vi "DAQNavi Write (Digital Wfm 1Chan 1Samp).vi"(8 "error in (no error)":errorcluster, 9 "timeout":dbl=10.0, 10 "data":digitalwaveform(waveform)={"t0"=timestamp(0 s since 1904-01-01), "dt"=1.0, "Y"={"transitions"=[], "data"=[]}}, 11 "task in":i32) -> (0 "error out":errorcluster, 2 "number of samples written per channel":u32, 3 "task out":i32)   [LabVIEW 2020]
uses:
  <vilib>/Waveform/DWDTOps.llb/DWDT Digital to Binary U8.vi
  DAQNavi_LV.dll
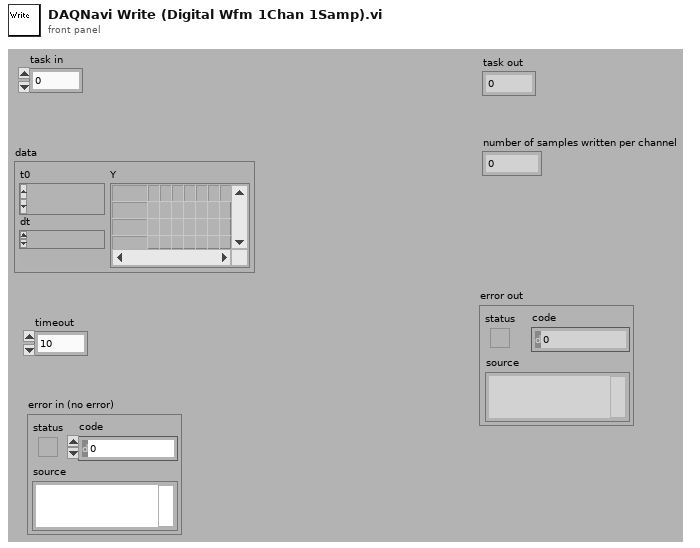
[diagram p1: front panel]
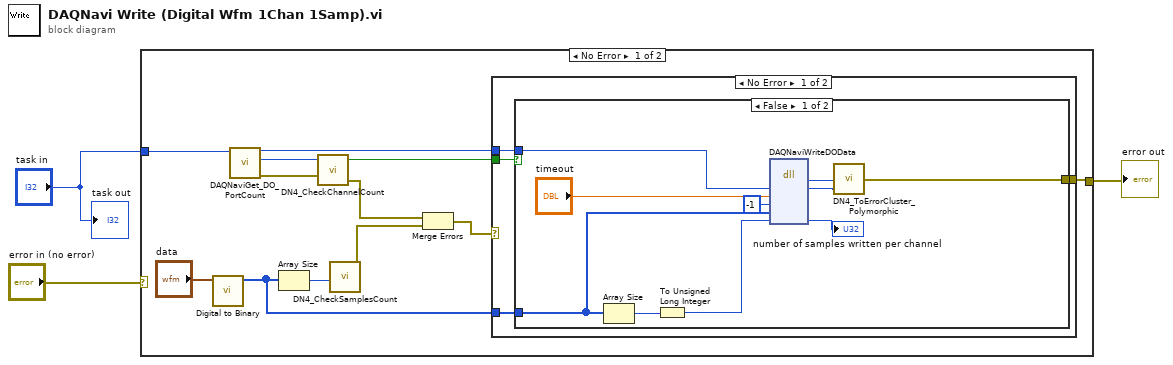
[diagram p0: block diagram]
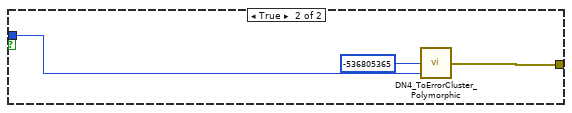
[diagram p2: hidden frame]
diagram:
  n1 = case shown="No Error" "error in (no error)" {
    selector: "error in (no error)" -> [_ w34]
    tunnel: [w14 w34] -> w2
    tunnel: "task in" -> [w15 _]
    frame No Error {
      n2 = call-poly <vilib>:"Digital to Binary.vi"("digital waveform"="data") -> ("binary array"=w4:u8[])  [unwired: 1 in, 9 out]
      n3 = call "DAQNaviGet_DO_PortCount.vi"("task in"=w15) -> ("error out"=w11:errorcluster, "port count"=w12:i32, "task out"=w10:i32)  [unwired: 1 in, 7 out]
      n4 = Array Size(array=w4) -> (size(s)=w6:i32)
      n5 = call "DN4_CheckChannelCount.vi"("error out"=w11, "channel count"=w12) -> ("error IO"=w8:errorcluster, "greater than 1?"=w9:bool)  [unwired: 2 out]
      n6 = call "DN4_CheckSamplesCount.vi"("samples count"=w6) -> ("error out"=w7:errorcluster)
      n7 = Merge Errors(w8, w7) -> (w13:errorcluster)
      n8 = case shown="No Error" w13 {
        selector: w13 -> [_ w33]
        tunnel: w9 -> [w19 _]
        tunnel: w10 -> [w18 _]
        tunnel: [w17 w33] -> w14
        tunnel: w4 -> [w16 _]
        frame No Error {
          n9 = case shown="False" w19 {
            tunnel: [w25 w31] -> w17
            tunnel: w18 -> [w29 w30]
            tunnel: w16 -> [w22 _]
            frame False {
              n10 = Array Size(array=w22) -> (size(s)=w24:i32)
              n11 = To Unsigned Long Integer(number=w24) -> (unsigned 32bit integer=w23:u32)
              n12 = dll-call lib="DAQNavi_LV.dll" fn="DAQNaviWriteDOData"("taskID"=w29, "timeout"="timeout", "portBit"=-1, "portData"=w22, "samples"=w23) -> ("return type"=w26:i32, "taskID"=w21:i32, "samples"=→"number of samples written per channel":u32)  [unwired: 6 in, 2 out]
              n13 = call "DN4_ToErrorCluster_Polymorphic.vi"("task id"=w21, "error code"=w26) -> ("error out"=w25:errorcluster)  [unwired: 3 out]
            }
            frame True {
              n14 = call "DN4_ToErrorCluster_Polymorphic.vi"("task id"=w30, "error code"=-536805365 ("error code (0)")) -> ("error out"=w31:errorcluster)  [unwired: 3 out]
            }
          }
        }
        frame Error {
        }
      }
    }
    frame Error {
    }
  }
  "error out" <- w2
  "task out" <- "task in"
